vi "Camera Joystick.vi"() -> ()   [LabVIEW 2016]
uses:
  Drivers/Aerotech A3200/Aerotech VIs.lvlib
panel:
  in  "Joystick":bool=TRUE
  in  "Stop":bool
  out "Image Out":T1(plugin-control)
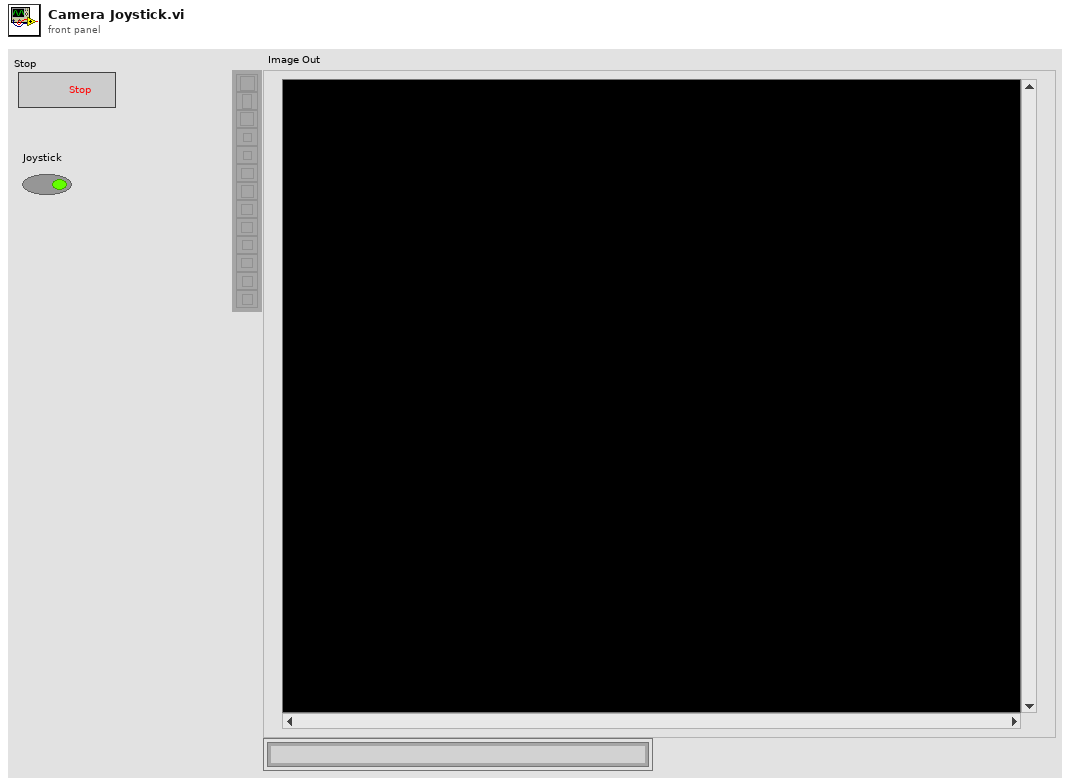
[diagram p1: front panel]
types:
  T1 = typedef "IMAQ Image.ctl" = refnum<image>
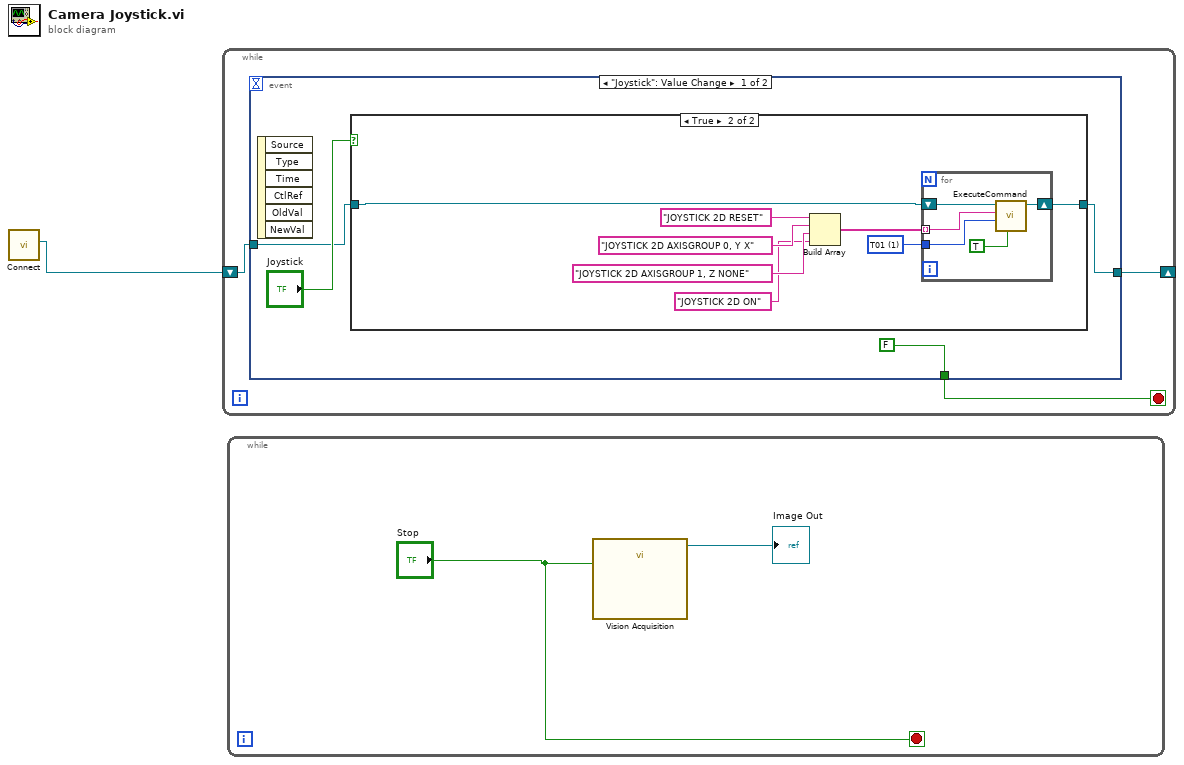
[diagram p0: block diagram]
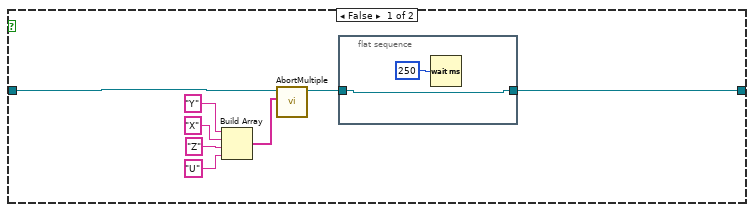
[diagram p2: hidden frame]
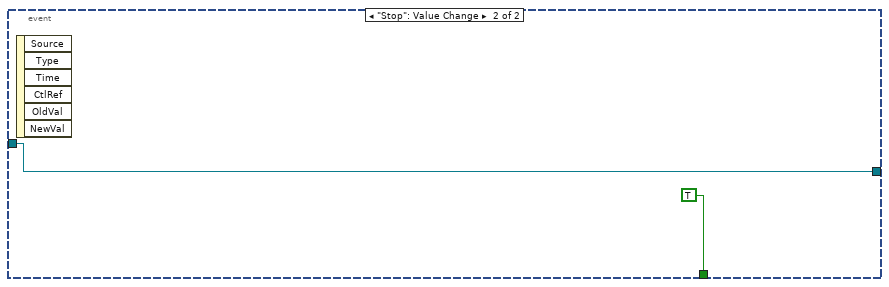
[diagram p3: hidden frame]
diagram:
  n1 = call "Connect.vi"() -> ("controller"=w1:refnum<k24>)  [unwired: 10 in, 1 out]
  n2 = while {
    shift-right: [w3] -> _
    shift-left: w1 -> [w4]
    stop <- w2 stop-if-true
    n3 = event shown="[0] \"Joystick\": Value Change" {
      selector: _ -> [_ _]
      dyn-events: _ -> [_ _]
      timeout: _ -> [_ _]
      tunnel: w4 -> [w7 w32]
      tunnel: [w6 w32] -> w3
      tunnel: [FALSE TRUE] -> w2
      event "Joystick": Value Change {
        n4 = event-data() -> ()  [unwired: 1 in, 6 out]
        n5 = case shown="True" "Joystick" {
          tunnel: w7 -> [w10 w20]
          tunnel: [w9 w19] -> w6
          frame False {
            n6 = Build Array("Y" ("axis name"), "X", "Z", "U") -> (w12:string[])
            n7 = call "AbortMultiple.vi"("axis names"=w12, "controller in"=w10) -> ("controller out"=w11:refnum<k24>)  [unwired: 8 in, 1 out]
            n8 = flat-sequence {
              tunnel: w11 -> [w18]
              tunnel: [w18] -> w9
              frame #0 {
                n9 = Wait (ms)(milliseconds to wait=u32 250) -> ()  [unwired: 1 out]
              }
            }
          }
          frame True {
            w22 = 1 items=["TLibrary", "T01", "T02", "T03", "T04", "T05", "T06", "T07", "T08", "T09", "T10", "T11", "T12", "T13", "T14", "T15", "T16", "T17", "T18", "T19", "T20", "T21", "T22", "T23", "T24", "T25", "T26", "T27", "T28", "T29", "T30", "T31"] ("taskId")
            n10 = Build Array("JOYSTICK 2D RESET", "JOYSTICK 2D AXISGROUP 0, Y X", "JOYSTICK 2D AXISGROUP 1, Z NONE", "JOYSTICK 2D ON") -> (w23:string[])
            n11 = for {
              tunnel: w23 -> [w31] mode=indexing
              tunnel: w22 -> [w30]
              shift-right: [w27] -> w19
              shift-left: w20 -> [w29]
              n12 = call "ExecuteCommand.vi"("return immediately"=TRUE, "taskId"=w30, "Command Code"=w31, "controller in"=w29) -> ("controller out"=w27:refnum<k24>)  [unwired: 5 in, 2 out]
            }
          }
        }
      }
      event "Stop": Value Change {
        n13 = event-data() -> ()  [unwired: 1 in, 6 out]
      }
    }
  }
  n14 = while {
    stop <- "Stop" stop-if-true
    n15 = call "Vision Acquisition"("Stop (F)"="Stop") -> ("Image Out"=→"Image Out":T1)  [unwired: 24 in, 2 out]
  }
